vi "Example Callback - DateTime Callback.vi"(4 "DateTime":refnum<user-event>, 5 "Event Data":T1, 6 "Control Ref":refnum<k24>, 7 "Event Common Data":T2) -> ()   [LabVIEW 2010]
uses:
  C:/tf/play/labview/Tinkerforge.dll
  Tinkerforge.dll
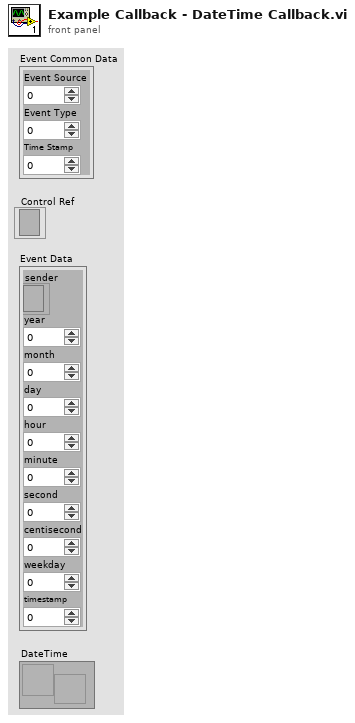
[diagram p1: front panel]
types:
  T1 = cluster{"sender":refnum<k24>, "year":i32, "month":u8, "day":u8, "hour":u8, "minute":u8, "second":u8, "centisecond":u8, "weekday":u8, "timestamp":i64}
  T2 = cluster{"Event Source":i32, "Event Type":u32, "Time Stamp":u32}
  T3 = cluster{"year":i32, "month":u8, "day":u8, "hour":u8, "minute":u8, "second":u8, "centisecond":u8, "weekday":u8, "timestamp":i64}
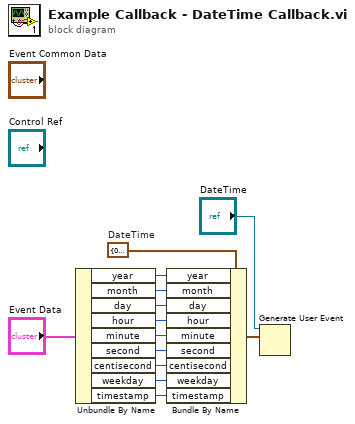
[diagram p0: block diagram]
diagram:
  w12 = T3 {"year"=0, "month"=0, "day"=0, "hour"=0, "minute"=0, "second"=0, "centisecond"=0, "weekday"=0, "timestamp"=0}  # DateTime
  n1 = Unbundle By Name("Event Data") -> ("year"=w11:i32, "month"=w10:u8, "day"=w9:u8, "hour"=w8:u8, "minute"=w7:u8, "second"=w6:u8, "centisecond"=w5:u8, "weekday"=w4:u8, "timestamp"=w3:i64)
  n2 = Bundle By Name(cluster=w12, "year"=w11, "month"=w10, "day"=w9, "hour"=w8, "minute"=w7, "second"=w6, "centisecond"=w5, "weekday"=w4, "timestamp"=w3) -> (w2:T3)
  n3 = Generate User Event(user event="DateTime", event data cluster=w2) -> ()  [unwired: 1 in, 2 out]
